vi "GT Get Control Config Ex.vi"(8 "error in (no error)":errorcluster caption="错误输入（无错误）", 9 "pControl":T1, 10 "control":i16, 11 "cardNum":i16) -> (0 "error out":errorcluster caption="错误输出", 1 "pControl out":T1, 3 "function return":i16)   [LabVIEW 2020, in "gts.lvlib"]
doc: "GT_API GT_GetControlConfigEx(short cardNum,short control,TControlConfigEx *pControl);"
uses:
  gts.lvlib
  dll/32bit/multi_card/gts.dll
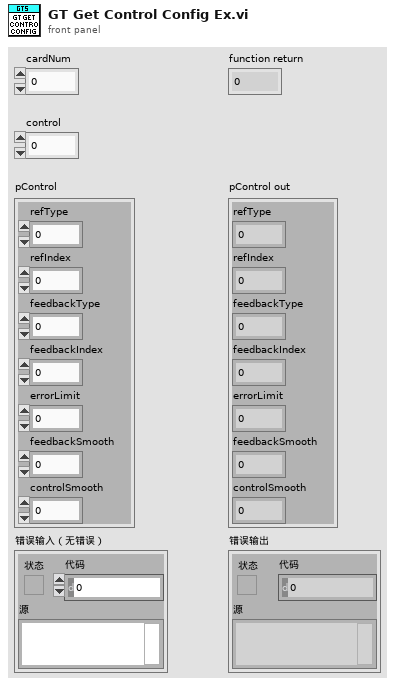
[diagram p1: front panel]
types:
  T1 = cluster{"refType":i16, "refIndex":i16, "feedbackType":i16, "feedbackIndex":i16, "errorLimit":i32, "feedbackSmooth":i16, "controlSmooth":i16}
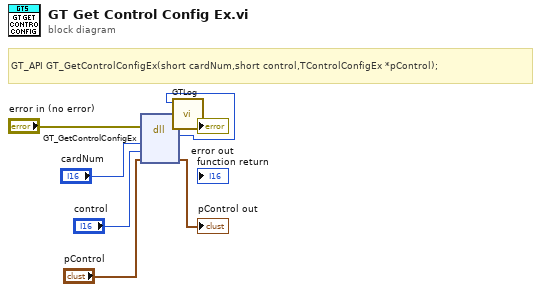
[diagram p0: block diagram]
diagram:
  # "GT_API GT_GetControlConfigEx(short cardNum,short control,TControlConfigEx *pControl);"
  n1 = dll-call lib="C:/1228/dll/32bit/multi_card/gts.dll" fn="GT_GetControlConfigEx"(error in="error in (no error)", "cardNum"="cardNum", "control"="control", "pControl"="pControl") -> (error out=w3:errorcluster, w1:i16, "pControl"=→"pControl out":T1)  [unwired: 4 in, 1 out]
  n2 = call "GTLog.vi"("error in (no error)"=w3, "Numeric"=w1) -> ("error out"=→"error out":errorcluster)  [unwired: 9 in]
